vi "Compare Images.vi"(8 "error in (no error)":errorcluster, 10 "Test Image Data":u32[][](array[numeric]), 11 "UUT Image Data":u32[][](array[numeric])) -> (0 "error out":errorcluster, 1 "Number of Dead Pixels":i32, 2 "Average Pixel Difference":dbl, 3 "UUT Image":picture)   [LabVIEW 2011]
uses:
  <vilib>/picture/picture.llb/Draw True-Color Pixmap.vi
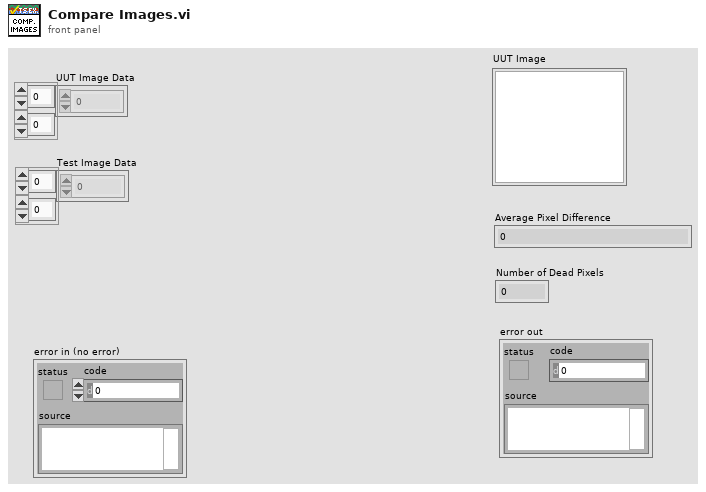
[diagram p1: front panel]
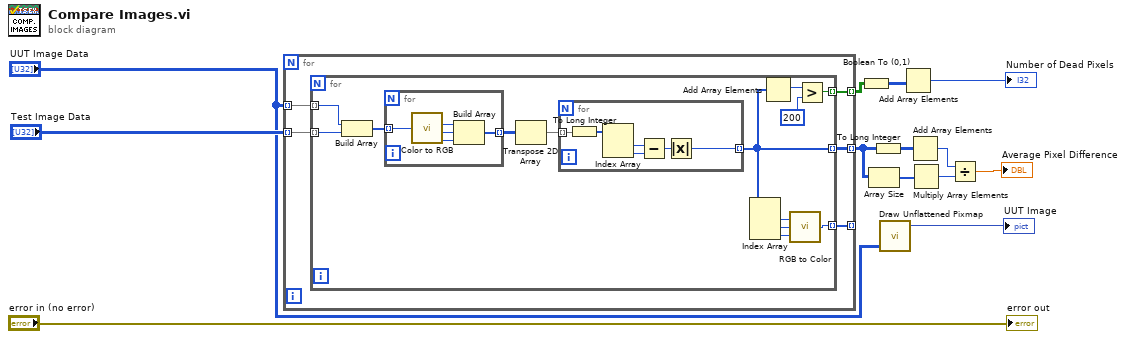
[diagram p0: block diagram]
diagram:
  n1 = for {
    tunnel: "Test Image Data" -> [w18] mode=indexing
    tunnel: "UUT Image Data" -> [w17] mode=indexing
    tunnel: [w16] -> w9 mode=indexing
    tunnel: [w15] -> _ mode=indexing
    tunnel: [w14] -> w6 mode=indexing
    n2 = for {
      tunnel: w18 -> [w27] mode=indexing
      tunnel: w17 -> [w28] mode=indexing
      tunnel: [w20] -> w16 mode=indexing
      tunnel: [w23] -> w15 mode=indexing
      tunnel: [w19] -> w14 mode=indexing
      n3 = Build Array(w28, w27) -> (w31:u32[])
      n4 = for {
        tunnel: w31 -> [w40] mode=indexing
        tunnel: [w39] -> w30 mode=indexing
        n5 = call <vilib>:"Color to RGB.vi"("Color"=w40) -> ("R"=w42:u8, "G"=w41:u8, "B"=w38:u8)  [unwired: 1 out]
        n6 = Build Array(w42, w41, w38) -> (w39:u8[])
      }
      n7 = Transpose 2D Array(2D array=w30) -> (transposed array=w29:u8[][])
      n8 = for {
        tunnel: [w32] -> w20 mode=indexing
        tunnel: w29 -> [w37] mode=indexing
        n9 = To Long Integer(number=w37) -> (32bit integer=w36:i32[])
        n10 = Index Array(array=w36) -> (element #1=w35:i32, element #2=w34:i32)  [unwired: 2 in]
        n11 = Subtract(x=w35, y=w34) -> (x-y=w33:i32)
        n12 = Absolute Value(x=w33) -> (abs(x)=w32:i32)
      }
      n13 = Index Array(array=w20) -> (element #1=w26:i32, element #2=w25:i32, element #3=w24:i32)  [unwired: 3 in]
      n14 = Add Array Elements(numeric array=w20) -> (sum=w21:i32)
      n15 = call <vilib>:"RGB to Color.vi"("B"=w24, "G"=w25, "R"=w26) -> ("Color"=w23:u32)
      n16 = Greater?(x=w21, y=200 ("x")) -> (0:w19:bool)
    }
  }
  n17 = Boolean To (0,1)(Boolean=w6) -> (0, 1=w5:i16[][])
  n18 = Array Size(array=w9) -> (size(s)=w11:i32[])
  n19 = To Long Integer(number=w9) -> (32bit integer=w8:i32[][][])
  n20 = call-poly <vilib>:"Draw Unflattened Pixmap.vi"("data (RGB format)"="UUT Image Data") -> ("new picture"=→"UUT Image":picture)  [unwired: 8 in]
  n21 = Add Array Elements(numeric array=w5) -> (sum=→"Number of Dead Pixels":i16)
  n22 = Add Array Elements(numeric array=w8) -> (sum=w13:i32)
  n23 = Multiply Array Elements(1:w11) -> (0:w10:i32)
  n24 = Divide(x=w13, y=w10) -> (x/y=→"Average Pixel Difference":dbl)
  "error out" <- "error in (no error)"
